vi "SubVI_Define_ROI_objeto.vi"(8 "error in (no error)":errorcluster, 10 "ROI Esteira":T5 {"Contours"."Type" items=["No Selection", "Point", "Line", "Rectangle", "Oval", "Polygon", "Free", "Annulus", "Unused2", "Unused3", "Broken Line", "Free Hand Line", "Rotated Rectangle"]}, 11 "Session In":T2) -> (0 "error out":errorcluster, 1 "ROI Objeto":T4 {"Contours"."Type" items=["No Selection", "Point", "Line", "Rectangle", "Oval", "Polygon", "Freehand Region", "Annulus", "Unused2", "Unused3", "Broken Line", "Freehand Line", "Rotated Rectangle"]}, 2 "Posição objeto":sgl[](array[numeric]), 3 "Session Out":T2)   [LabVIEW 2017]
uses:
  <vilib>/userdefined/High Color/IMAQdx.ctl
  <vilib>/vision/driver/IMAQdx.llb/IMAQdx Buffer Number Mode.ctl
  <vilib>/vision/driver/NI_Vision_Acquisition_Software.lvlib
  <vilib>/vision/NI_Vision_Development_Module.lvlib
panel:
  out "Objects":T1(array[cluster]) {"Aspect Ratio" format="%.2f"; "Orientation" format="%.2f"; "Area" format="%.2f"; "Object Center"."Y" format="%.2f"; "Object Center"."X" format="%.2f"}
  out "Number of Objects":i32
  out "Imagem Original":T3(plugin-control)
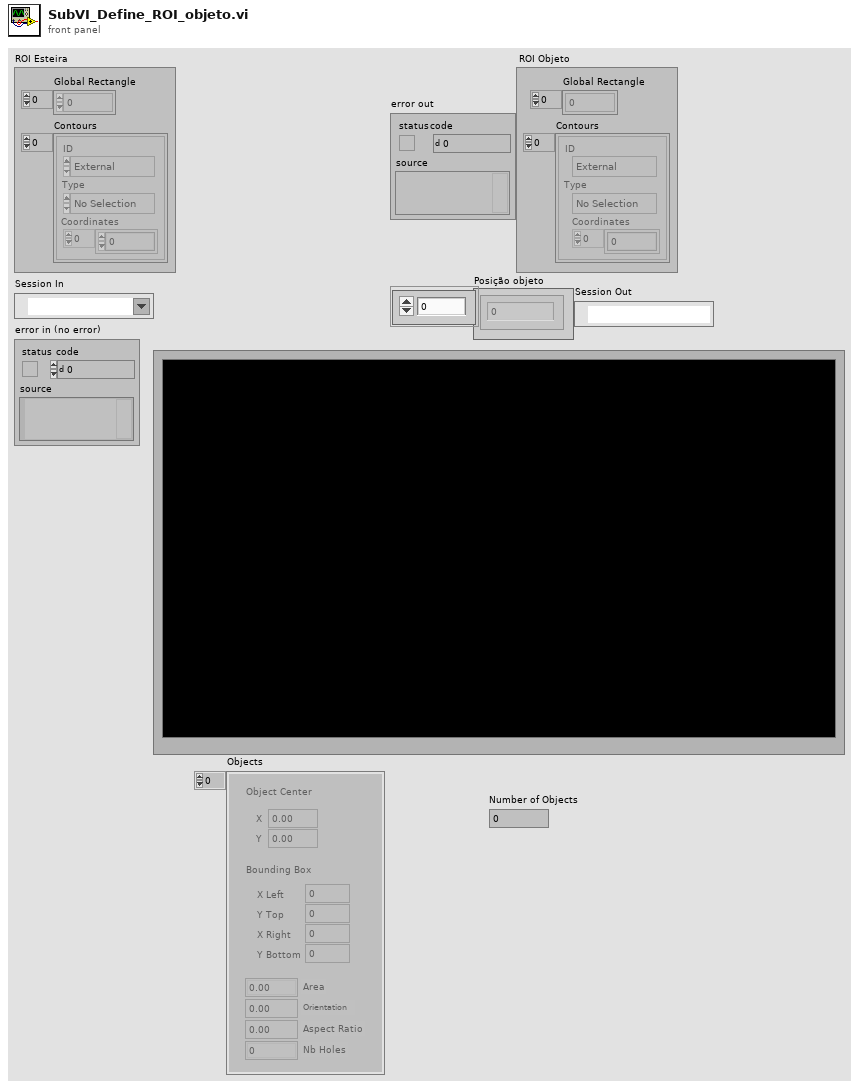
[diagram p1: front panel]
types:
  T1 = cluster{"Object Center":cluster{"X":sgl, "Y":sgl}, "Bounding Box":cluster{"X Left":i32, "Y Top":i32, "X Right":i32, "Y Bottom":i32}, "Area":sgl, "Orientation":sgl, "Aspect Ratio":sgl, "Nb Holes":i32}[]
  T2 = typedef "IMAQdx.ctl" = refnum<k21>
  T3 = typedef "IMAQ Image.ctl" = refnum<image>
  T4 = typedef "ROI Descriptor" = cluster{"Global Rectangle":i32[], "Contours":cluster{"ID":enum32{"External", "Internal"}, "Type":u32, "Coordinates":i32[]}[]}
  T5 = cluster{"Global Rectangle":i32[], "Contours":cluster{"ID":enum32{"External", "Internal"}, "Type":u32, "Coordinates":i32[]}[]}
  T6 = cluster{"Objects":u16, "Threshold":i32, "Reject Border":bool, "Fill Holes":bool, "Min Object Size":bool, "Min Size":i32, "Max Object Size":bool, "Max Size":i32, "Show Search Area":bool, "Show Center":bool, "Show Bounding Box":bool}
  T7 = typedef "NI_Vision_Acquisition_Software.lvlib/IMAQdx Buffer Number Mode.ctl" = enum32{"Next", "Last", "Buffer Number", "Every", "Last New"}
  T8 = typedef "Image Type" = u32
  T9 = typedef "IMAQ Rectangle" = cluster{"Left":i32, "Top":i32, "Right":i32, "Bottom":i32, "Rotation":dbl}
  T10 = cluster{"Object Center":cluster{"X":sgl, "Y":sgl}, "Bounding Box":cluster{"X Left":i32, "Y Top":i32, "X Right":i32, "Y Bottom":i32}, "Area":sgl, "Orientation":sgl, "Aspect Ratio":sgl, "Nb Holes":i32}
  T11 = cluster{"X Left":i32, "Y Top":i32, "X Right":i32, "Y Bottom":i32}
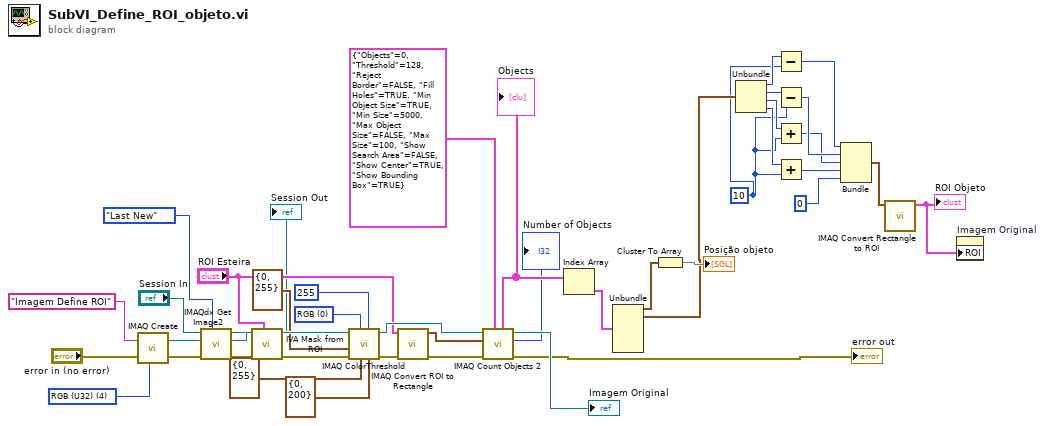
[diagram p0: block diagram]
diagram:
  w6 = 10
  w36 = u16 0 items=["RGB", "HSL", "HSV", "HSI"] ("Color Mode")
  w42 = T8 4 items=["Grayscale (U8)", "Grayscale (I16)", "Grayscale (SGL)", "Complex (CSG)", "RGB (U32)", "HSL (U32)", "RGB (U64)", "Grayscale (U16)"] ("Image Type")
  n1 = call "IMAQ Create"("Image Name"="Imagem Define ROI", "Image Type"=w42, "error in (no error)"="error in (no error)") -> ("New Image"=w40:T3, "error out"=w39:errorcluster)  [unwired: 2 in]
  n2 = call <vilib>:"IMAQdx Get Image2.vi"("Buffer Number Mode (Next)"=IMAQdx_Buffer_Number_Mode."Last New", "error in"=w39, "Image In"=w40, "Session In"="Session In") -> ("error out"=w23:errorcluster, "Image Out"=w38:T3, "Session Out"=→"Session Out":T2)  [unwired: 4 in, 1 out]
  n3 = call <vilib>:"IVA Mask from ROI.vi"("ROI Descriptor"="ROI Esteira", "error in (no error)"=w23, "Image Src"=w38) -> ("error out"=w22:errorcluster, "Image Out"=w37:T3)  [unwired: 2 in, 5 out]
  n4 = call "IMAQ ColorThreshold"("Blue or Luma or Val or Inten Range"=cluster{"Lower value":i32, "Upper value":i32} {"Lower value"=0, "Upper value"=200}, "Replace Value"=255, "Green or Sat Range"=cluster{"Lower value":i32, "Upper value":i32} {"Lower value"=0, "Upper value"=255}, "Color Mode"=w36, "error in (no error)"=w22, "Red or Hue Range"=cluster{"Lower value":i32, "Upper value":i32} {"Lower value"=0, "Upper value"=255}, "Image Src"=w37) -> ("error out"=w21:errorcluster, "Image Dst Out"=w29:T3)  [unwired: 1 in, 2 out]
  n5 = call "IMAQ Convert ROI to Rectangle"("error in (no error)"=w21, "ROI Descriptor"="ROI Esteira") -> ("error out"=w20:errorcluster, "Rectangle"=w30:T9)  [unwired: 7 in]
  n6 = call "IMAQ Count Objects 2"("Settings"=T6 {"Objects"=0, "Threshold"=128, "Reject Border"=FALSE, "Fill Holes"=TRUE, "Min Object Size"=TRUE, "Min Size"=5000, "Max Object Size"=FALSE, "Max Size"=100, "Show Search Area"=FALSE, "Show Center"=TRUE, "Show Bounding Box"=TRUE}, "error in (no error)"=w20, "Search Rect (entire image)"=w30, "Image"=w29) -> ("error out"=→"error out":errorcluster, "Number of Objects"=→"Number of Objects":i32, "Image Out"=→"Imagem Original":T3, "Objects"=w28:T1)  [unwired: 3 in, 1 out]
  "Objects" <- w28
  n7 = Index Array(array=w28) -> (element=w27:T10)  [unwired: 1 in]
  n8 = Unbundle(w27) -> ("Object Center"=w17:cluster{"X":sgl, "Y":sgl}, "Bounding Box"=w15:T11)  [unwired: 4 out]
  n9 = Cluster To Array(cluster=w17) -> (array=→"Posição objeto":sgl[])
  n10 = Unbundle(w15) -> ("X Left"=w13:i32, "Y Top"=w11:i32, "X Right"=w14:i32, "Y Bottom"=w12:i32)
  n11 = Subtract(x=w13, y=w6) -> (x-y=w10:i32)
  n12 = Subtract(x=w11, y=w6) -> (x-y=w9:i32)
  n13 = Add(x=w14, y=w6) -> (x+y=w8:i32)
  n14 = Add(x=w12, y=w6) -> (x+y=w7:i32)
  n15 = Bundle(w10, w9, w8, w7, 0) -> (w18:cluster{i32, i32, i32, i32, i32})  [unwired: 1 in]
  n16 = call "IMAQ Convert Rectangle to ROI"("Rectangle"=w18) -> ("ROI Descriptor"=w3:T4)  [unwired: 8 in, 1 out]
  "ROI Objeto" <- w3
  n17 = property on="Imagem Original" class="ImageControl"("ROI"=w3) -> ()  [unwired: 2 in, 2 out]
